vi "XGB 연속 읽기.vi"() -> ()   [LabVIEW 2014]
uses:
  <vilib>/Instr/_visa.llb/VISA Configure Serial Port (Instr).vi
panel:
  out "U16배열":u16[](array[numeric])=[4096, 8192, 12288, 16384, 20480, 24576, 28672, 32768, 36864, 40960, 0, 0, 0, 0, 0, 0, 0, 0, 0, 0, 0, 0, 0, 0, 0, 0, 0, 0, 0, 0, 0, 0, 0, 0, 0, 0, 0, 0, 0, 0, 0, 0, 0, 0, 0, 0, 0, 0, 0, 0]
  in  "VISA resource name":refnum<visa-resource-name>="COM4"
  out "error out":errorcluster={"status"=FALSE, "code"=1073676294, "source"="XGB 연속 읽기.vi 안에 VISA 읽기"} caption="에러 출력"
  out "응답 프레임":string="\u000600RSB0164100020003000400050006000700080009000A0000000000000000000000000000000000000000000000000000000000000000000000000000000000000000000000000000000000000000000000000000000000000000000000000000000000000000000\u0003"
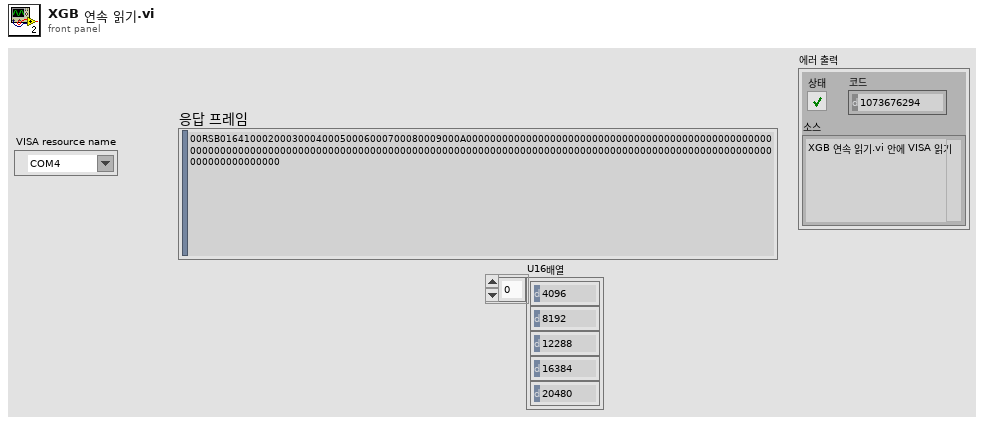
[diagram p1: front panel]
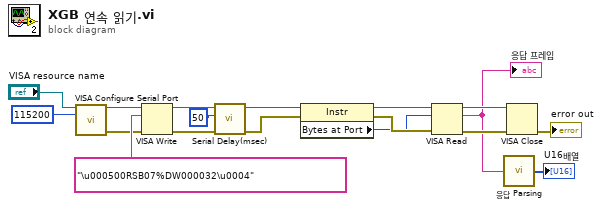
[diagram p0: block diagram]
diagram:
  n1 = call-poly "VISA Configure Serial Port"("VISA resource name"="VISA resource name", "baud rate (9600)"=u32 115200 ("baud rate")) -> ("VISA resource name out"=w8:refnum<visa-resource-name>, "error out"=w7:errorcluster)  [unwired: 12 in]
  n2 = VISA Write(VISA resource name=w8, write buffer="\u000500RSB07%DW000032\u0004" ("요구 프레임"), error in (no error)=w7) -> (VISA resource name out=w15:refnum<visa-resource-name>, error out=w12:errorcluster)  [unwired: 1 out]
  n3 = call "Serial Delay(msec).vi"("에러 입력(에러 없음)"=w12, "milliseconds to wait"=u32 50, "VISA 참조 번호 입력"=w15) -> ("에러 출력"=w13:errorcluster, "VISA 참조 번호 출력"=w14:refnum<visa-resource-name>)  [unwired: 7 in]
  n4 = property class="Instr"(reference=w14, error in=w13) -> (reference out=w16:refnum<visa-resource-name>, error out=w17:errorcluster, "Bytes at Port"=w3:u32)
  n5 = VISA Read(VISA resource name=w16, byte count=w3, error in (no error)=w17) -> (VISA resource name out=w6:refnum<visa-resource-name>, read buffer=w2:string, error out=w5:errorcluster)  [unwired: 1 out]
  "응답 프레임" <- w2
  n6 = call "응답 Parsing.vi"("응답 프레임"=w2) -> ("U16배열"=→"U16배열":u16[])
  n7 = VISA Close(VISA resource name=w6, error in (no error)=w5) -> (error out=→"error out":errorcluster)
